vi "Input Files.vi"(8 "error in (no error)":errorcluster) -> (0 "error out":errorcluster)   [LabVIEW 2009]
uses:
  lib/MixedMode/Widget/Input File Step Actions.ctl
  lib/Data Access Objects/Metadata/Persistant DAO Actions.ctl
panel:
  in  "Ok":bool
  in  "LBCB 2 Input File":path
  in  "LBCB 1 Input File":path
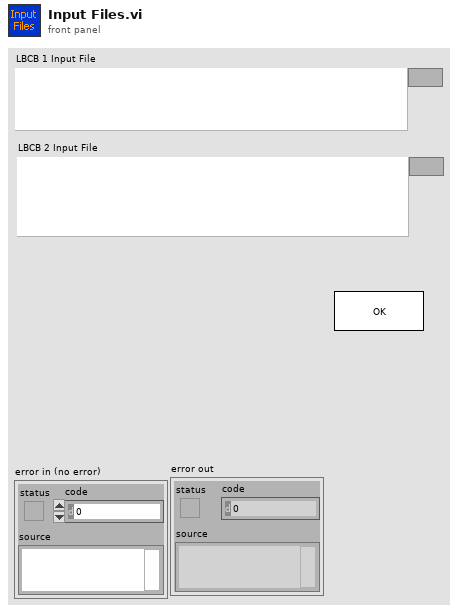
[diagram p1: front panel]
types:
  T1 = typedef "Persistant DAO Actions.ctl" = enum16{"Init", "Get", "Set", "Load", "Save"}
  T2 = typedef "Input File Step Actions.ctl" = enum16{"Load", "Next Step", "Reset", "Get Step"}
  T3 = typedef "Number Of LBCBs.ctl" = enum16{"1", "2"}
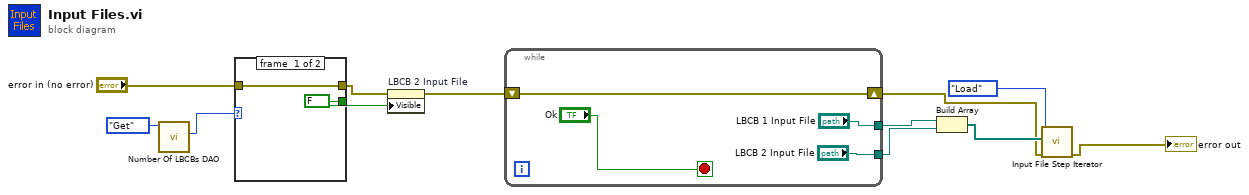
[diagram p0: block diagram]
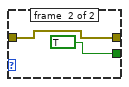
[diagram p2: hidden frame]
diagram:
  n1 = call "Number Of LBCBs DAO.vi"("Actions"=Persistant_DAO_Actions."Get") -> ("Number of\nLBCBs Out"=w7:T3)  [unwired: 8 in, 2 out]
  n2 = case shown="\"2\"" w7 {
    tunnel: [FALSE ("Visible") TRUE ("Visible")] -> w6
    tunnel: "error in (no error)" -> [w13 w15]
    tunnel: [w13 w15] -> w3
    frame #0 {
    }
    frame #1 {
    }
  }
  n3 = property on="LBCB 2 Input File" class="Path"(error in=w3, "Visible"=w6) -> (error out=w5:errorcluster)  [unwired: 1 in, 1 out]
  n4 = while {
    tunnel: ["LBCB 1 Input File"] -> w10
    tunnel: ["LBCB 2 Input File"] -> w9
    shift-right: [w17] -> w2
    shift-left: w5 -> [w17]
    stop <- "Ok" stop-if-true
  }
  n5 = Build Array(w10, w9) -> (w11:path[])
  n6 = call "Input File Step Iterator.vi"("error in (no error)"=w2, "LBCB Input Files"=w11, "Input File Step Actions"=Input_File_Step_Actions."Load") -> ("error out"=→"error out":errorcluster)  [unwired: 3 in, 3 out]
